vi "FourierTransform.vi"() -> ()   [LabVIEW 2013]
panel:
  in  "F":dbl caption="Frequencia"
  in  "n":dbl(slide)=1.0 caption="Harmonicas" min=1.0 max=10000.0 step=1.0 scale=0.0..100.0
  out "Harmonicas":cluster{"X":dbl[], "Y":dbl[]}[](graph)
  out "Sinal":cluster{dbl[], dbl[]}(graph)
  in  "dt":dbl caption="Precisao temporal (dt)"
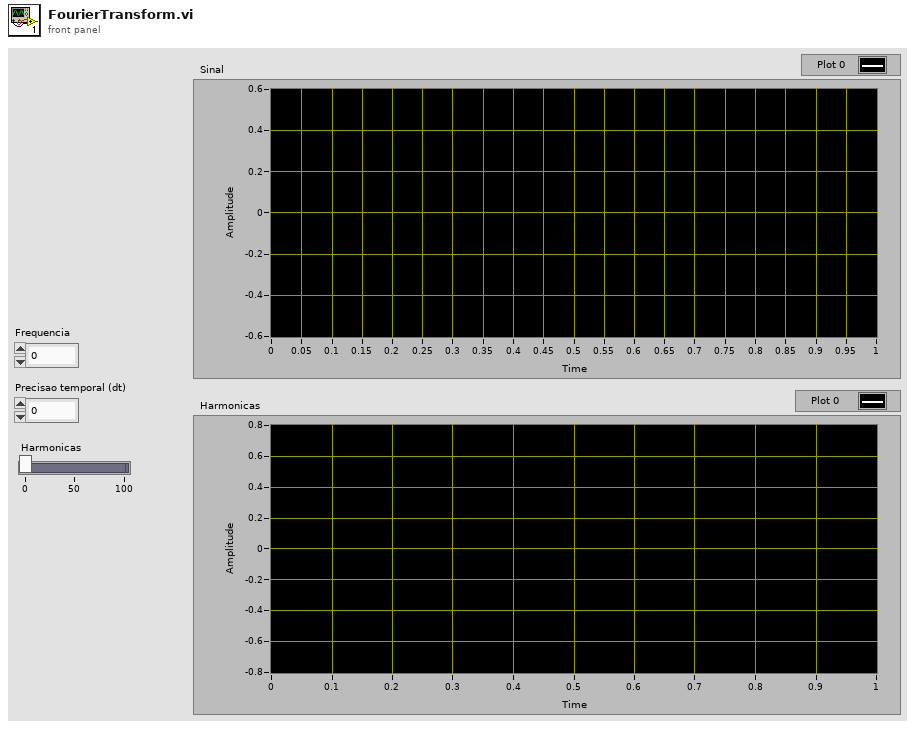
[diagram p1: front panel]
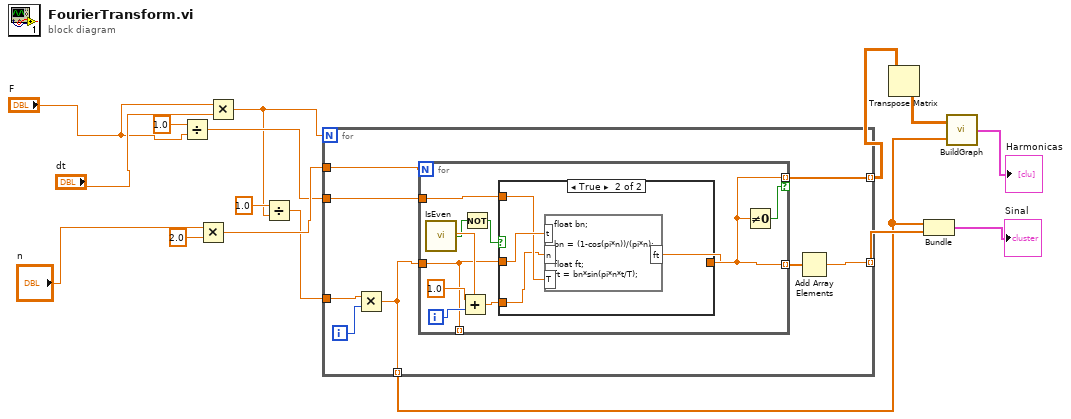
[diagram p0: block diagram]
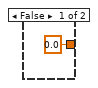
[diagram p2: hidden frame]
diagram:
  n1 = Divide(x=1.0, y="F") -> (x/y=w9:dbl)
  n2 = Multiply(x="n", y=2.0) -> (x*y=w13:dbl)
  n3 = Multiply(x="F", y="dt") -> (x*y=w7:dbl)
  n4 = Divide(x=1.0, y=w7) -> (x/y=w6:dbl)
  n5 = for {
    N: w7 -> [_]
    tunnel: w13 -> [w23]
    tunnel: w9 -> [w22]
    tunnel: [w20] -> w16 mode=indexing
    tunnel: [w19] -> w5 mode=indexing
    tunnel: [w18] -> w12 mode=indexing
    tunnel: w6 -> [w17]
    i -> [w24]
    n6 = Multiply(x=w17, y=w24) -> (x*y=w19:dbl)
    n7 = for {
      N: w23 -> [_]
      tunnel: [w25] -> w21 mode=indexing
      tunnel: w19 -> [w29]
      tunnel: w22 -> [w30]
      tunnel: [w29] -> _ mode=indexing
      tunnel: [w25] -> w18 mode=indexing if=w26
      i -> [w33]
      n8 = Add(x=1.0, y=w33) -> (x+y=w31:dbl)
      n9 = call "IsEven.vi"("Numeric"=w31) -> ("Boolean"=w28:bool)
      n10 = Not(x=w28) -> (.not. x?=w27:bool)
      n11 = case shown="True" w27 {
        tunnel: [0.0 w36] -> w25
        tunnel: w31 -> [_ w35]
        tunnel: w29 -> [_ w38]
        tunnel: w30 -> [_ w37]
        frame False {
        }
        frame True {
          n12 = formula code="float bn;\n\nbn = (1-cos(pi*n))/(pi*n);\n\nfloat ft;\nft = bn*sin(pi*n*t/T);"("t"=w38, "n"=w35, "T"=w37) -> ("ft"=w36:dbl)
        }
      }
      n13 = Not Equal To 0?(x=w25) -> (x != 0?=w26:bool)
    }
    n14 = Add Array Elements(numeric array=w21) -> (sum=w20:dbl)
  }
  n15 = Transpose Matrix(1:w12) -> (0:w4:dbl[][])
  n16 = Bundle(w5, w16) -> (→"Sinal":cluster{dbl[], dbl[]})  [unwired: 1 in]
  n17 = call "BuildGraph.vi"("X"=w5, "Y"=w4) -> ("Graph"=→"Harmonicas":cluster{"X":dbl[], "Y":dbl[]}[])
